vi "Queue Caller.vi"(9 "Priority?":bool, 10 "Msg":refnum<class "Msg.lvclass">, 11 "jettl Event Actor in":refnum<class "jettl Event Actor.lvclass">) -> (3 "jettl Event Actor out":refnum<class "jettl Event Actor.lvclass">)   [LabVIEW 2021, in "jettl Event Actor.lvlib" / "jettl Event Actor.lvclass"]
uses:
  Actor/Msg/Msg.lvclass
  jettl Event Actor.lvclass
  jettl Event Actor.lvclass/jettl Event Actor.ctl
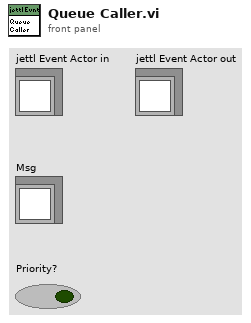
[diagram p1: front panel]
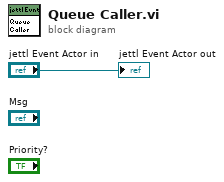
[diagram p0: block diagram]
diagram:
  "jettl Event Actor out" <- "jettl Event Actor in"
